vi "Serial.vi"() -> ()   [LabVIEW 2013]
uses:
  <vilib>/Instr/_visa.llb/VISA Configure Serial Port (Instr).vi
  <vilib>/ptbypt/NI_PtbyPt.lvlib
panel:
  in  "Res. de shunt (ohm)":dbl
  in  "Área do núcleo (m^2)":dbl
  in  "Comp. do enrolamento (m)":dbl
  in  "Espiras do secundário":dbl
  in  "Espiras do primário":dbl
  in  "Res. interador (kOhm)":dbl
  in  "Cap. integrador (uF)":dbl
  out "Campo Magnético":dbl(graph)
  out "FFT Fluxo":dbl[](graph)
  out "FFT Campo Magnético":dbl[](graph)
  out "Laço de histerese":cluster{dbl[], dbl[]}(graph)
  in  "Chart History":i32=500 caption="Amostras"
  in  "stop 2":bool
  out "Fluxo":dbl(graph)
  in  "Baud rate":u32=9600
  in  "Porta COM":refnum<visa-resource-name>
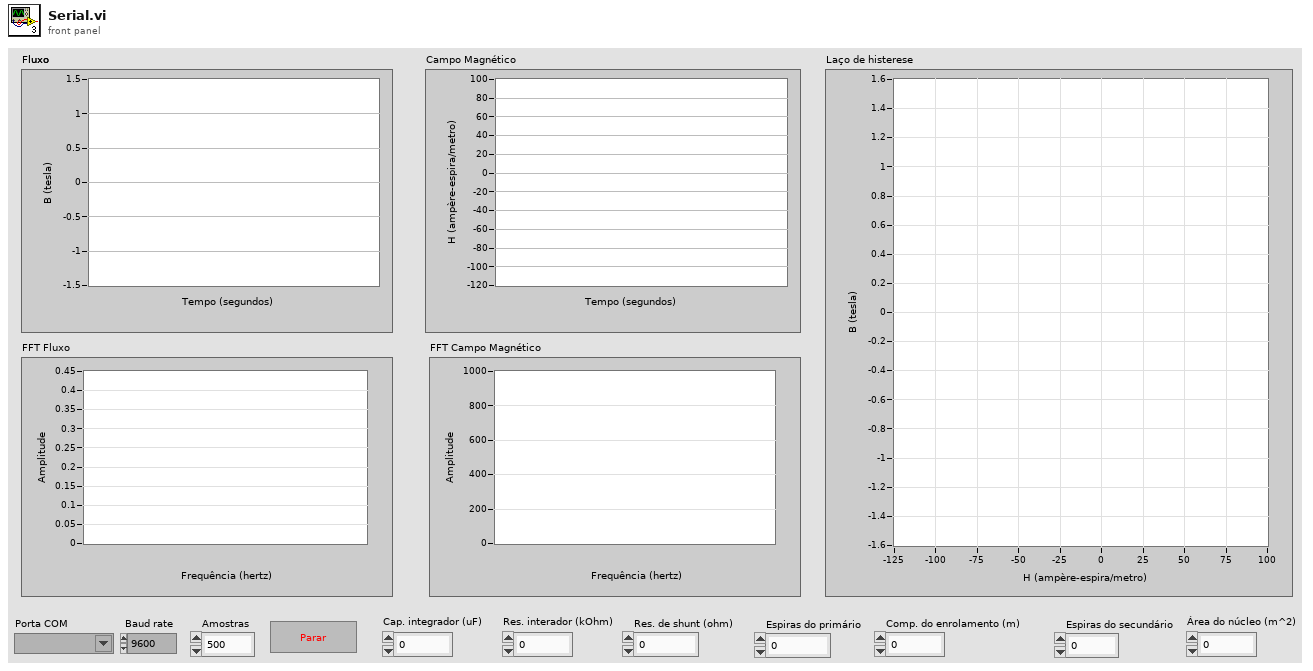
[diagram p1: front panel]
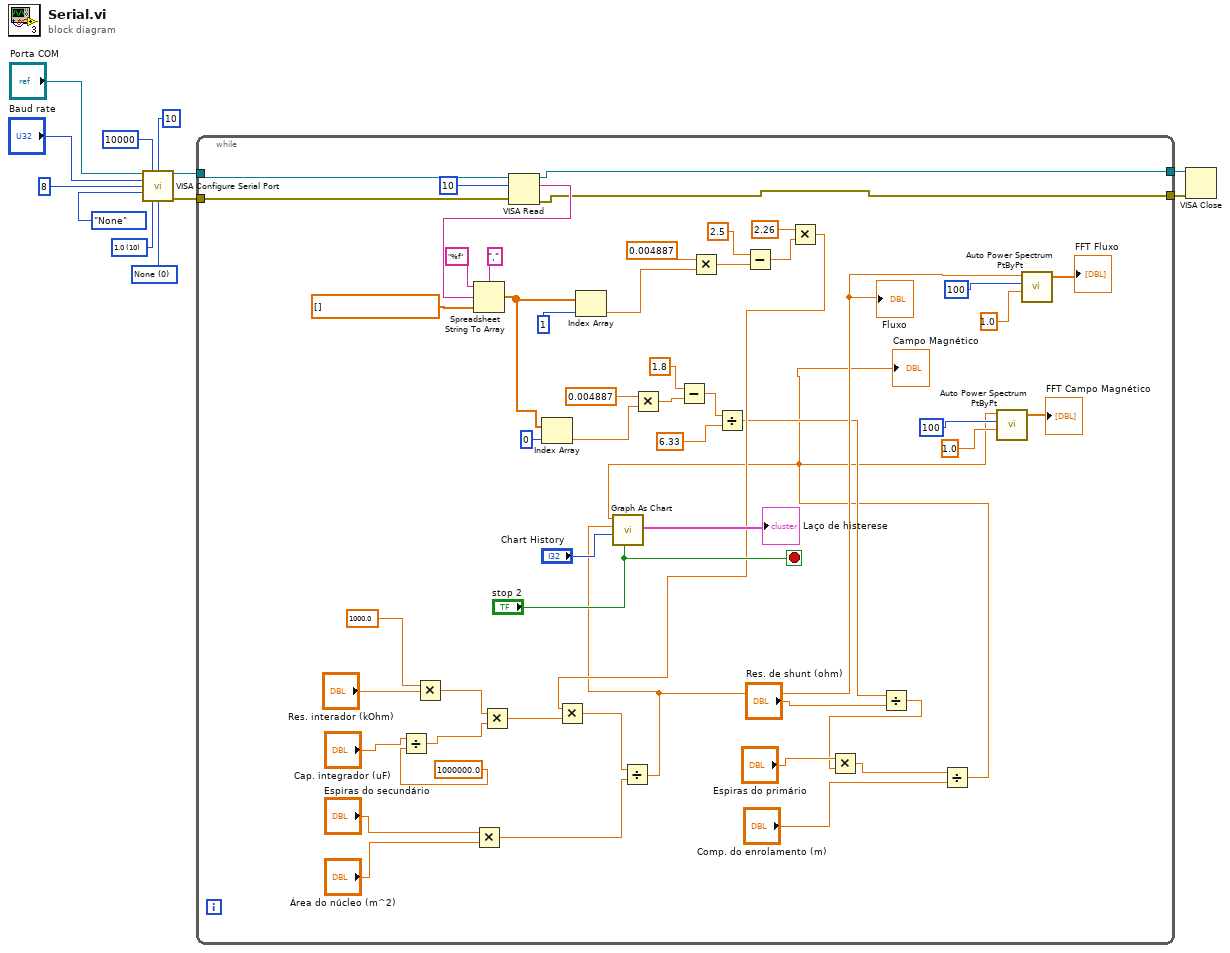
[diagram p0: block diagram]
diagram:
  w5 = u16 0 items=["None", "XON/XOFF", "RTS/CTS", "XON/XOFF & RTS/CTS", "DTR/DSR", "XON/XOFF & DTR/DSR"] ("flow control (0:none)")
  w6 = u16 10 items=["1.0"=10, "1.5"=15, "2.0"=20] ("stop bits (10: 1 bit)")
  n1 = call-poly "VISA Configure Serial Port"("VISA resource name"="Porta COM", "timeout (10sec)"=u32 10000, "termination char\n(0xA = '\\n' = LF)"=u8 10 ("termination char\n(0xA = '\\n' = LF)"), "baud rate (9600)"="Baud rate", "data bits (8)"=u16 8, "parity (0:none)"=enum16{"None", "Odd", "Even", "Mark", "Space"}."None", "stop bits (10: 1 bit)"=w6, "flow control (0:none)"=w5) -> ("VISA resource name out"=w11:refnum<visa-resource-name>, "error out"=w2:errorcluster)  [unwired: 6 in]
  n2 = while {
    tunnel: w11 -> [w59]
    tunnel: [w65] -> w10
    tunnel: w2 -> [w58]
    tunnel: [w52] -> w1
    stop <- "stop 2" stop-if-true
    n3 = Divide(x="Cap. integrador (uF)", y=1000000.0 ("x")) -> (x/y=w33:dbl)
    n4 = Multiply(x=1000.0, y="Res. interador (kOhm)") -> (x*y=w34:dbl)
    n5 = Multiply(x="Espiras do secundário", y="Área do núcleo (m^2)") -> (x*y=w26:dbl)
    n6 = Multiply(x=w34, y=w33) -> (x*y=w30:dbl)
    n7 = VISA Read(VISA resource name=w59, byte count=u32 10, error in (no error)=w58) -> (VISA resource name out=w65:refnum<visa-resource-name>, read buffer=w64:string, error out=w52:errorcluster)  [unwired: 1 out]
    n8 = Spreadsheet String To Array(delimiter (Tab)=",", format string="%f", spreadsheet string=w64, array type (2D Dbl)=dbl[] []) -> (array=w56:dbl[])
    n9 = Index Array(array=w56, index=0 ("index (row)")) -> (element=w37:dbl)
    n10 = Index Array(array=w56, index=1 ("index (row)")) -> (element=w38:dbl)
    n11 = Multiply(x=0.004887, y=w37) -> (x*y=w40:dbl)
    n12 = Subtract(x=1.8, y=w40) -> (x-y=w21:dbl)
    n13 = Multiply(x=0.004887, y=w38) -> (x*y=w39:dbl)
    n14 = Divide(x=w21, y=6.33) -> (x/y=w17:dbl)
    n15 = Subtract(x=2.5, y=w39) -> (x-y=w29:dbl)
    n16 = Multiply(x=2.26, y=w29) -> (x*y=w25:dbl)
    n17 = Multiply(x=w25, y=w30) -> (x*y=w27:dbl)
    n18 = Divide(x=w27, y=w26) -> (x/y=w24:dbl)
    "Fluxo" <- w24
    n19 = Divide(x=w17, y="Res. de shunt (ohm)") -> (x/y=w16:dbl)
    n20 = Multiply(x="Espiras do primário", y=w16) -> (x*y=w14:dbl)
    n21 = Divide(x=w14, y="Comp. do enrolamento (m)") -> (x/y=w15:dbl)
    "Campo Magnético" <- w15
    n22 = call "Graph As Chart.vi"("Clear Graph?"="stop 2", "Chart History (10,000)"="Chart History", "Y Value"=w24, "X Value"=w15) -> ("XY Graph"=→"Laço de histerese":cluster{dbl[], dbl[]})  [unwired: 7 in]
    n23 = call <vilib>:"Auto Power Spectrum PtByPt.vi"("signal"=w15, "sample length"=100, "dt"=1.0) -> ("Power Spectrum (V^2 rms)"=→"FFT Campo Magnético":dbl[])  [unwired: 2 in, 2 out]
    n24 = call <vilib>:"Auto Power Spectrum PtByPt.vi"("signal"=w24, "sample length"=100, "dt"=1.0) -> ("Power Spectrum (V^2 rms)"=→"FFT Fluxo":dbl[])  [unwired: 2 in, 2 out]
  }
  n25 = VISA Close(VISA resource name=w10, error in (no error)=w1) -> ()  [unwired: 1 out]
